vi "WriteToConnection.vi"(8 "error in (no error)":errorcluster, 10 "Setpoints to boat":T1, 11 "TCP Small Boat in":refnum<class "TCP Small Boat.lvclass">) -> (0 "error out":errorcluster, 3 "TCP Small Boat out":refnum<class "TCP Small Boat.lvclass">)   [LabVIEW 2011, in "TCP Small Boat.lvclass"]
uses:
  TCP Small Boat.lvclass
  2-RIO/2 Typedefs/setpoints to boat.ctl
  2-RIO/2 Typedefs/sail setpt.ctl
  2-RIO/2 Typedefs/rudder angle.ctl
panel:
  out "Output Array":u8[](array[numeric])
  out "Setpoints to boat out":T1
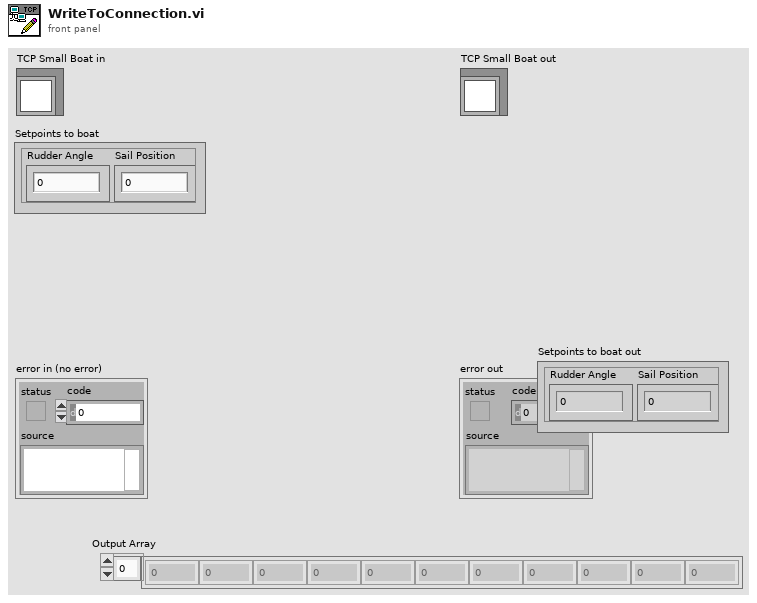
[diagram p1: front panel]
types:
  T1 = typedef "setpoints to boat.ctl" = cluster{"Sail Position":T2, "Rudder Angle":T3}
  T2 = typedef "sail setpt.ctl" = dbl
  T3 = typedef "rudder angle.ctl" = dbl
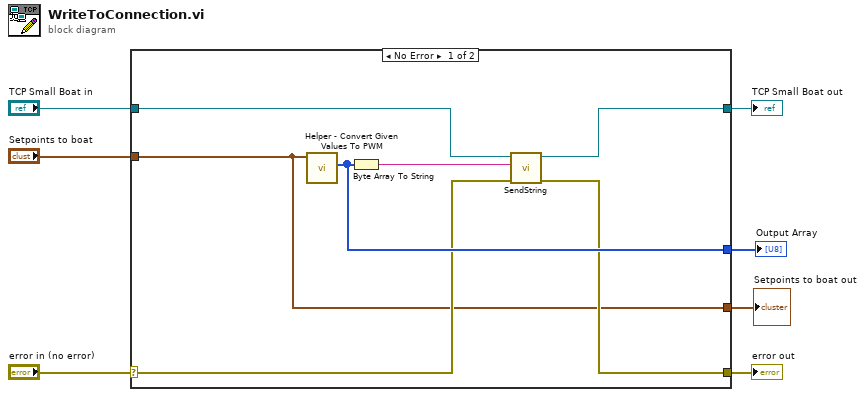
[diagram p0: block diagram]
diagram:
  n1 = case shown="No Error" "error in (no error)" {
    selector: "error in (no error)" -> [w12 w16]
    tunnel: [w10 w16] -> w6
    tunnel: [w9 w15] -> w4
    tunnel: "TCP Small Boat in" -> [w13 w15]
    tunnel: [w8 _] -> w3
    tunnel: [w14 _] -> w2
    tunnel: "Setpoints to boat" -> [w8 _]
    frame No Error {
      n2 = call "Helper - Convert Given Values To PWM.vi"("Setpoints to boat"=w8) -> ("Output Array, integers"=w14:u8[])  [unwired: 9 in, 1 out]
      n3 = Byte Array To String(unsigned byte array=w14) -> (string=w11:string)
      n4 = call-dynamic "SendString.vi"("error in (no error)"=w12, "data in"=w11, "TCP Connection in"=w13) -> ("error out"=w10:errorcluster, "TCP Connection out"=w9:refnum<class "TCP Small Boat.lvclass">)  [unwired: 6 in, 1 out]
    }
    frame Error {
    }
  }
  "error out" <- w6
  "TCP Small Boat out" <- w4
  "Setpoints to boat out" <- w3
  "Output Array" <- w2
